vi "Nonlinear Curve Fit Intervals.vi"(0 "Y":dbl[](array[numeric]), 1 "confidence level":dbl=0.95, 2 "f(x,a)":T1, 3 "data":variant, 5 "X":dbl[](array[numeric]), 7 "Weight":dbl[](array[numeric]), 9 "best fit parameters":dbl[](array[numeric]), 11 "error in (no error)":errorcluster) -> (4 "Upper Bound":dbl[](array[numeric]), 6 "Lower Bound":dbl[](array[numeric]), 10 "delta best fit parameters":dbl[](array[numeric]), 15 "error out":errorcluster)   [LabVIEW 2020, in "NI_Gmath.lvlib"]
doc: "Calculates statistical intervals of the best nonlinear fit for a data set (<B>X</B>, <B>Y</B>)."
uses:
  NI_Gmath.lvlib
  LM model function reference.ctl
  LM_output select.ctl
  Real A x B.vi
  Student t Inverse CDF.vi
  Real Inverse Matrix.vi
  NI_AALPro.lvlib
  NI_AALBase.lvlib
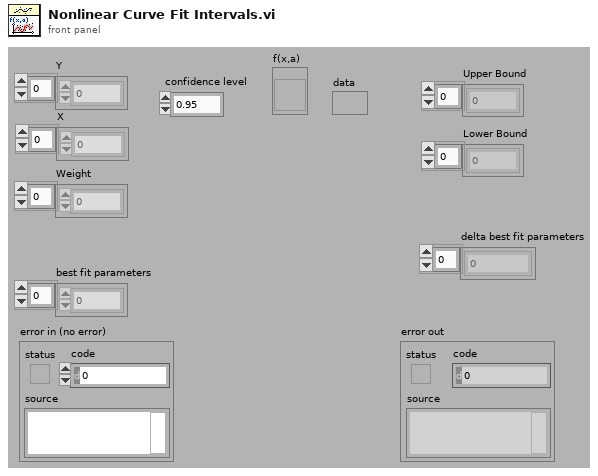
[diagram p1: front panel]
types:
  T1 = typedef "NI_Gmath.lvlib/LM model function reference.ctl" = refnum<vi>
  T2 = typedef "NI_Gmath.lvlib/LM_output select.ctl" = cluster{"model function":bool, "gradient":bool}
  T3 = typedef "NI_Matrix.lvlib/RealMatrix.ctl" = dbl[][]
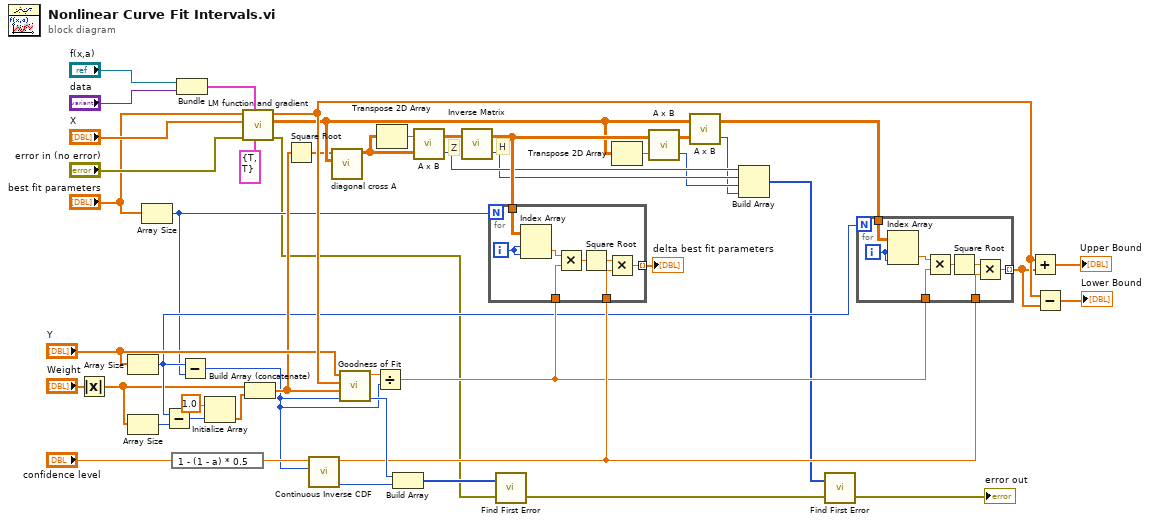
[diagram p0: block diagram]
diagram:
  # "H"
  # "Z"
  n1 = Absolute Value(x="Weight") -> (abs(x)=w4:dbl[])
  n2 = Array Size(array="Y") -> (size(s)=w14:i32)
  n3 = Array Size(array=w4) -> (size(s)=w21:i32)
  n4 = Array Size(array="best fit parameters") -> (size(s)=w13:i32)
  n5 = Subtract(x=w14, y=w21) -> (x-y=w18:i32)
  n6 = expression code="1 - (1 - a) * 0.5"("confidence level") -> (w34:dbl)
  n7 = Bundle("f(x,a)"="f(x,a)", "data"="data") -> (w44:cluster{"f(x,a)":T1, "data":variant})  [unwired: 1 in]
  n8 = Subtract(x=w14, y=w13) -> (x-y=w15:i32)
  n9 = Initialize Array(1.0, w18) -> (w20:dbl[])
  n10 = call "LM function and gradient.vi"("output control"=T2 {"model function"=TRUE, "gradient"=TRUE}, "model function"=w44, "error in (no error)"="error in (no error)", "X"="X", "a"="best fit parameters") -> ("error out"=w5:errorcluster, "gradient"=w3:dbl[][], "f(X)"=w26:dbl[])  [unwired: 3 in, 1 out]
  n11 = Build Array (concatenate)(w4, w20) -> (w16:dbl[])
  n12 = Square Root(x=w16) -> (sqrt(x)=w2:dbl[])
  n13 = call-poly "Continuous Inverse CDF.vi"("k degrees of freedom"=w15, "cdf(x)"=w34) -> ("error"=w33:i32, "x"=w28:dbl)  [unwired: 8 in]
  n14 = call "diagonal cross A.vi"("A"=w3, "diagonal"=w2) -> ("diagonalxA"=w1:T3)  [unwired: 9 in]
  n15 = call "Goodness of Fit.vi"("degree of freedom"=w15, "Weight"=w16, "Best Fit"=w26, "Y"="Y") -> ("error"=w36:i32, "SSE"=w37:dbl)  [unwired: 4 in, 2 out]
  n16 = Divide(x=w37, y=w15) -> (x/y=w23:dbl)
  n17 = Transpose 2D Array(2D array=w1) -> (transposed array=w40:T3)
  n18 = Build Array(w36, w33) -> (w35:i32[])
  n19 = call-poly "A x B.vi"("B"=w1, "A"=w40) -> ("error"=w12:i32, "A x B"=w39:T3)
  n20 = call-poly "Inverse Matrix.vi"("Input Matrix"=w39) -> ("error"=w11:i32, "Inverse Matrix"=w31:T3)  [unwired: 1 in]
  n21 = for {
    N: w13 -> [_]
    tunnel: w31 -> [w56]
    tunnel: w28 -> [w49]
    tunnel: [w53] -> w48 mode=indexing
    tunnel: w23 -> [w50]
    i -> [w55]
    n22 = Index Array(array=w56, index (row)=w55, index (col)=w55) -> (element=w51:dbl)
    n23 = Multiply(x=w51, y=w50) -> (x*y=w54:dbl)
    n24 = Square Root(x=w54) -> (sqrt(x)=w52:dbl)
    n25 = Multiply(x=w52, y=w49) -> (x*y=w53:dbl)
  }
  "delta best fit parameters" <- w48
  n26 = call "Find First Error.vi"("error in (no error)"=w5, "error codes"=w35) -> ("error out"=w8:errorcluster)  [unwired: 2 in, 1 out]
  n27 = Transpose 2D Array(2D array=w3) -> (transposed array=w32:dbl[][])
  n28 = call-poly "A x B.vi"("B"=w32, "A"=w31) -> ("error"=w10:i32, "A x B"=w30:T3)
  n29 = call-poly "A x B.vi"("B"=w30, "A"=w3) -> ("error"=w9:i32, "A x B"=w29:T3)
  n30 = Build Array(w12, w11, w10, w9) -> (w6:i32[])
  n31 = call "Find First Error.vi"("error in (no error)"=w8, "error codes"=w6) -> ("error out"=→"error out":errorcluster)  [unwired: 2 in, 1 out]
  n32 = for {
    N: w14 -> [_]
    tunnel: w29 -> [w64]
    tunnel: w28 -> [w62]
    tunnel: [w61] -> w25 mode=indexing
    tunnel: w23 -> [w59]
    i -> [w57]
    n33 = Index Array(array=w64, index (row)=w57, index (col)=w57) -> (element=w60:dbl)
    n34 = Multiply(x=w60, y=w59) -> (x*y=w58:dbl)
    n35 = Square Root(x=w58) -> (sqrt(x)=w63:dbl)
    n36 = Multiply(x=w63, y=w62) -> (x*y=w61:dbl)
  }
  n37 = Add(x=w26, y=w25) -> (x+y=→"Upper Bound":dbl[])
  n38 = Subtract(x=w26, y=w25) -> (x-y=→"Lower Bound":dbl[])
